vi "StopDataListener.vi"(0 "Connection ID":u64, 2 "ms timeout (-1)":i32=-1, 5 "error in (no error)":errorcluster) -> (19 "error out":errorcluster)   [LabVIEW 2014, in "FrontPanelPublisher.lvlib" / "Websocket.lvclass"]
uses:
  Websocket.lvclass
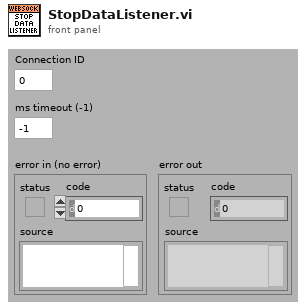
[diagram p1: front panel]
types:
  T1 = enum16{"ReadRepository", "CreateNew", "CreateOrLookUpExisting", "ReadRepositoryAndDestroy"}
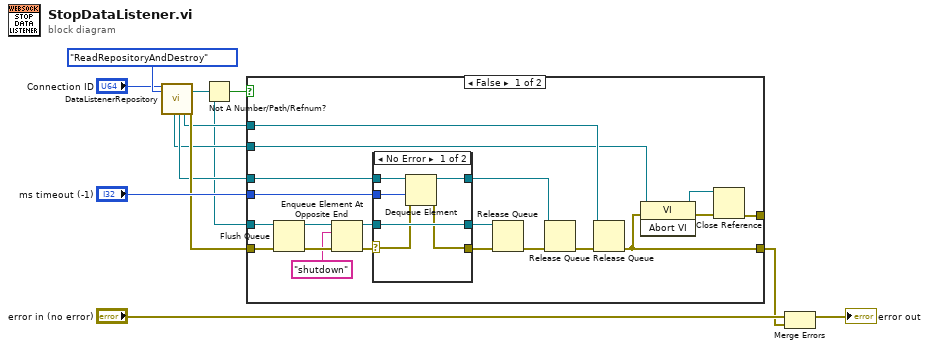
[diagram p0: block diagram]
diagram:
  n1 = call "DataListenerRepository.vi"("Connection ID"="Connection ID", "Action(ReadRepository)"=T1."ReadRepositoryAndDestroy") -> ("ProcessViRef"=w5:refnum<vi>, "ProcessSyncQueue"=w7:refnum<queue>, "FromProcessQueue"=w6:refnum<queue>, "ToProcessQueue"=w4:refnum<queue>, "error out"=w8:errorcluster)  [unwired: 12 in, 1 out]
  n2 = Not A Number/Path/Refnum?(number/path/refnum=w4) -> (NaN/Path/Refnum?=w3:bool)
  n3 = case shown="False" w3 {
    tunnel: w7 -> [w27 _]
    tunnel: w8 -> [w29 w42]
    tunnel: [w14 w42] -> w10
    tunnel: w4 -> [w32 _]
    tunnel: "ms timeout (-1)" -> [w23 _]
    tunnel: w6 -> [w21 _]
    tunnel: w5 -> [w16 _]
    tunnel: [w13 _] -> _
    frame False {
      n4 = Flush Queue(queue=w32, error in (no error)=w29) -> (queue out=w30:refnum<queue>, error out=w31:errorcluster)  [unwired: 1 out]
      n5 = Enqueue Element At Opposite End(queue=w30, element="shutdown", error in (no error)=w31) -> (queue out=w26:refnum<queue>, error out=w22:errorcluster)  [unwired: 1 in, 1 out]
      n6 = case shown="No Error" w22 {
        tunnel: [w34 w41] -> w25
        tunnel: w27 -> [w37 w39]
        tunnel: [w38 w40] -> w24
        tunnel: w26 -> [w38 w40]
        tunnel: w23 -> [w36 _]
        selector: w22 -> [w35 w41]
        tunnel: [w33 w39] -> w19
        frame No Error {
          n7 = Dequeue Element(queue=w37, timeout in ms (-1)=w36, error in (no error)=w35) -> (queue out=w33:refnum<queue>, error out=w34:errorcluster)  [unwired: 2 out]
        }
        frame Error {
        }
      }
      n8 = Release Queue(queue=w24, error in (no error)=w25) -> (error out=w20:errorcluster)  [unwired: 1 in, 2 out]
      n9 = Release Queue(queue=w19, error in (no error)=w20) -> (error out=w18:errorcluster)  [unwired: 1 in, 2 out]
      n10 = Release Queue(queue=w21, error in (no error)=w18) -> (error out=w14:errorcluster)  [unwired: 1 in, 2 out]
      n11 = invoke class="VI" method="Abort VI"(reference=w16, error in=w14) -> (reference out=w15:refnum<vi>, error out=w17:errorcluster)  [unwired: 1 in, 1 out]
      n12 = Close Reference(reference=w15, error in (no error)=w17) -> (error out=w13:errorcluster)
    }
    frame True {
    }
  }
  n13 = Merge Errors("error in (no error)", w10) -> (→"error out":errorcluster)
